vi "INTELLIFAUCET Start.vi"(4 "Refnum in":T1, 6 "Debug":bool, 8 "Error In":errorcluster, 10 "mS wait":u32=250, 11 "VISA session":refnum<visa-resource-name>="MW100") -> (0 "Error Out":errorcluster, 3 "dup VISA session":refnum<visa-resource-name>)   [LabVIEW 2016]
uses:
  MW100/Type Definitions/HEWH MW100 Channel Numbers.ctl
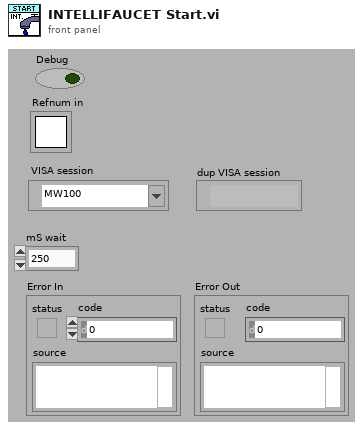
[diagram p1: front panel]
types:
  T1 = typedef "Semaphore RefNum" = refnum<k1>
  T2 = typedef "HEWH MW100 Channel Numbers.ctl" = string
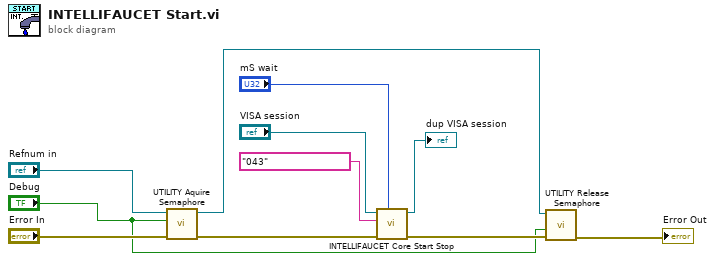
[diagram p0: block diagram]
diagram:
  n1 = call "UTILITY Aquire Semaphore.vi"("error in (no error)"="Error In", "Debug"="Debug", "Refnum in"="Refnum in") -> ("error out"=w6:errorcluster, "Refnum out"=w3:T1)  [unwired: 6 in, 1 out]
  n2 = call "INTELLIFAUCET Core Start Stop.vi"("mS wait"="mS wait", "error in (no error)"=w6, "HEWH MW100 Channel Numbers"=T2 "043", "VISA Refnum in"="VISA session") -> ("error out"=w5:errorcluster, "VISA Refnum out"=→"dup VISA session":refnum<visa-resource-name>)  [unwired: 6 in]
  n3 = call "UTILITY Release Semaphore.vi"("error in (no error)"=w5, "Debug"="Debug", "Refnum in"=w3) -> ("error out"=→"Error Out":errorcluster)  [unwired: 8 in]
